vi "ControlePosicaoServo2.vi"() -> ()   [LabVIEW 2012]
uses:
  <vilib>/LabVIEW Interface for Arduino/Type Defs/Board Type.ctl
  <vilib>/LabVIEW Interface for Arduino/Type Defs/Pin Mode.ctl
  <vilib>/Utility/file.llb/Read From Spreadsheet File (I64).vi
  <vilib>/LabVIEW Interface for Arduino/LabVIEW Interface for Arduino.lvlib
panel:
  out "?":cluster{"Referencia":dbl, "Atual":dbl}(graph)
  in  "Limpar Arquivo":bool
  in  "Gravar Posição KNOOB":bool
  out "Index":u32
  out "Comeco do Timer 2":i32
  in  "Comeco do Timer":i32
  in  "Ligar Controle":bool
  out "Voltage":dbl(knob) scale=0.0..5.0
  out "Sequencia":i64[](array[numeric])
  in  "Comeco do Arquivo":i32
  out "Elemento do Arquivo":i64
  in  "file path (dialog if empty)":path
  in  "TXT    KNOOB":bool
  out "PWM2":i32
  out "PWM1":i32
  out "Erro":dbl
  in  "Referencia":dbl(knob) scale=0.0..180.0
  out "Referencia":dbl(knob) scale=0.0..180.0
  in  "stop":bool
  out "Atual":dbl(knob) scale=0.0..180.0
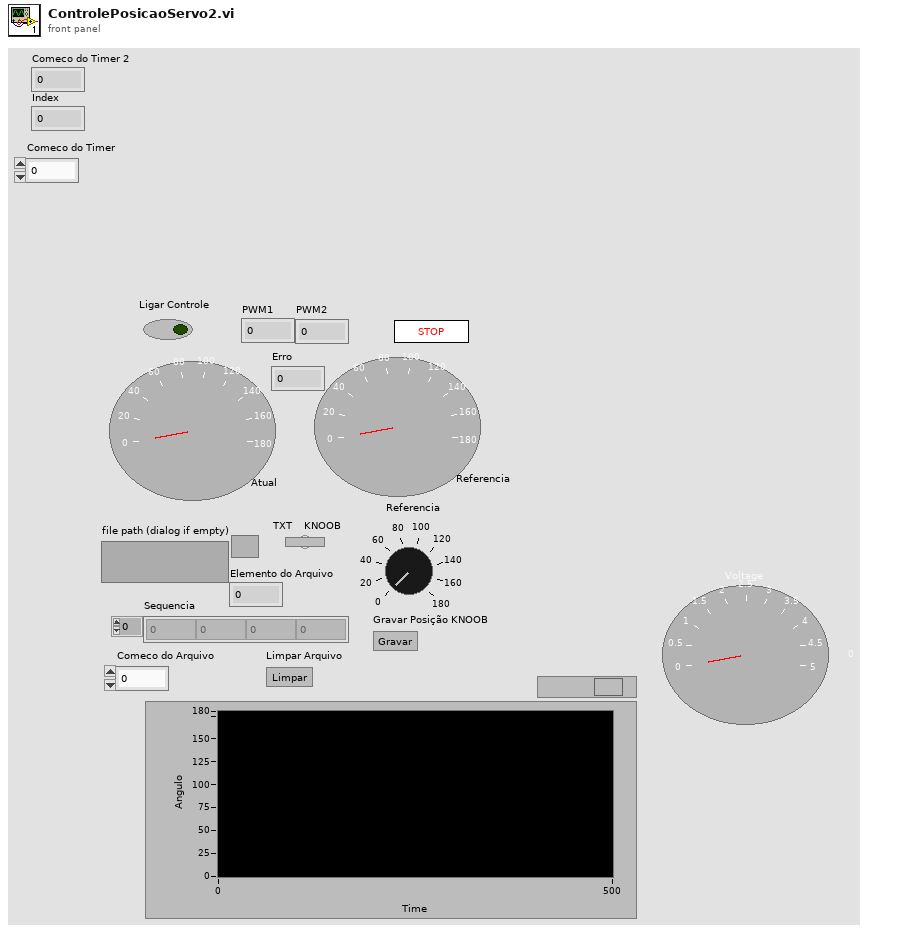
[diagram p1: front panel]
types:
  T1 = typedef "LabVIEW Interface for Arduino.lvlib/Board Type.ctl" = enum16{"Uno", "Dimuelanove w/Atmega 328", "Mega 2560"}
  T2 = typedef "LabVIEW Interface for Arduino.lvlib/Arduino Resource.ctl" = cluster{"VISA resource":refnum<visa-resource-name>, "Board Type":T1, "Connection Type":enum8{"USB / Serial"}, "Bytes Per Packet (15)":u8}
  T3 = typedef "LabVIEW Interface for Arduino.lvlib/Pin Mode.ctl" = enum8{"Input", "Output"}
  T4 = enum16{"open", "replace", "create", "open or create", "replace or create", "replace or create with confirmation"}
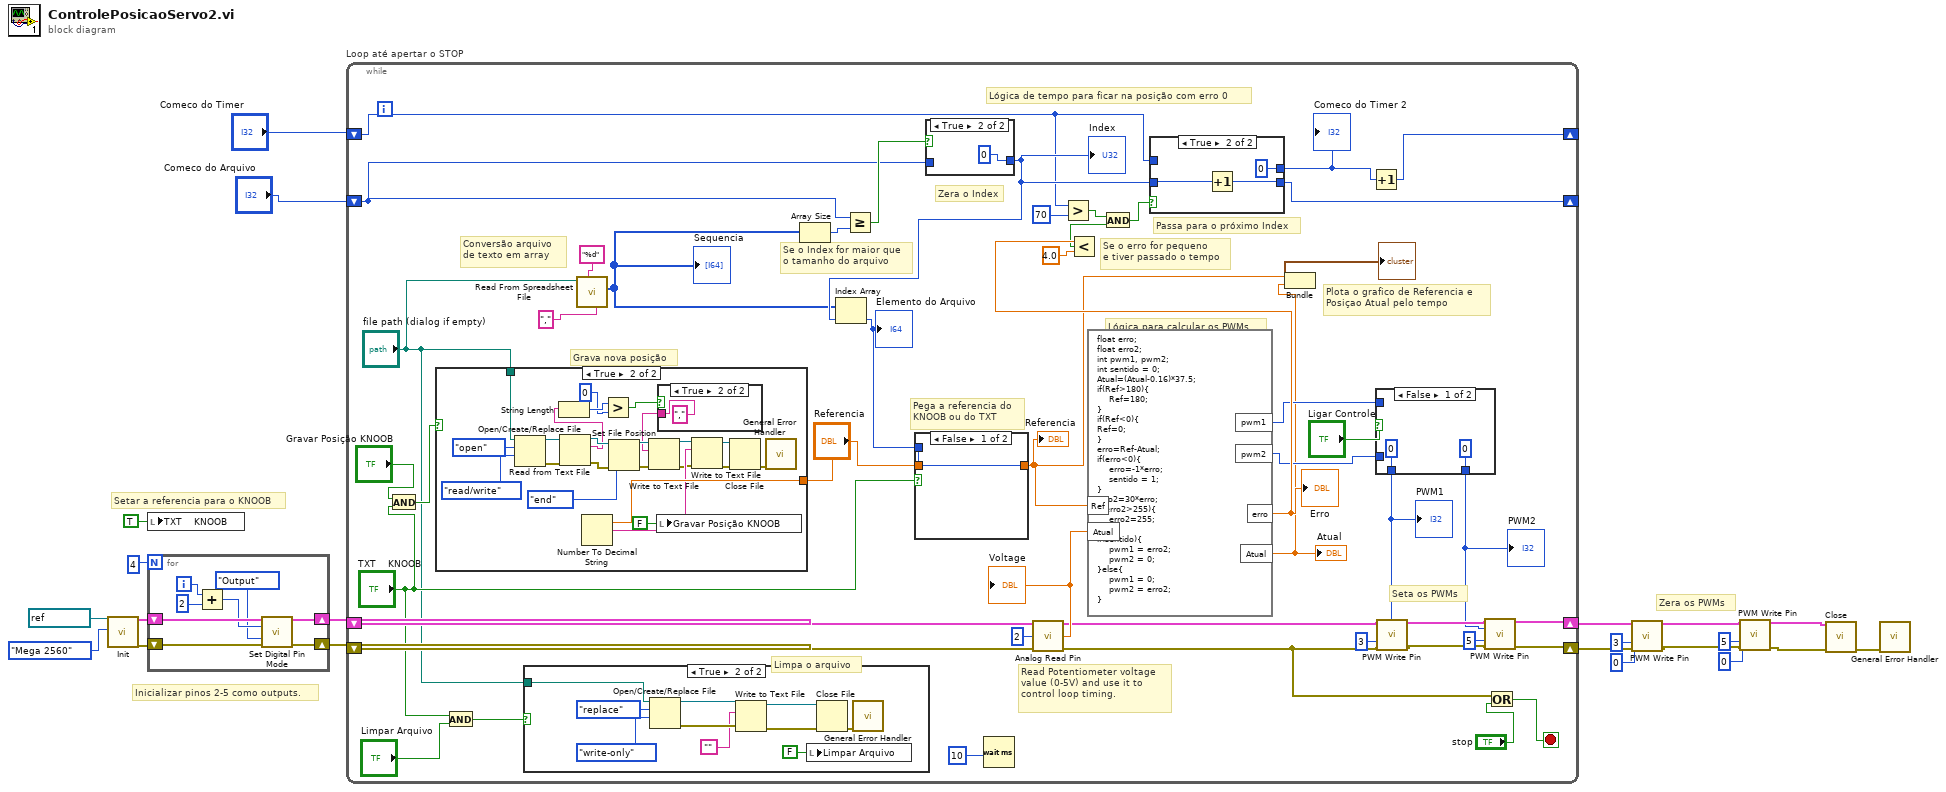
[diagram p0: block diagram]
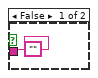
[diagram p4: hidden frame]
diagram:
  # "Zera os PWMs"
  # "Setar a referencia para o KNOOB"
  # "Inicializar pinos 2-5 como outputs."
  n1 = call <vilib>:"Init.vi"("VISA resource"=refnum<visa-resource-name> "COM6", "Board Type (Uno)"=Board_Type."Mega 2560") -> ("Arduino Resource"=w20:T2, "error out"=w21:errorcluster)  [unwired: 16 in]
  n2 = local write "TXT    KNOOB"(TRUE ("TXT    KNOOB")) -> ()
  n3 = for {
    N: 4 -> [_]
    shift-right: [w27] -> w19
    shift-left: w20 -> [w28]
    shift-right: [w26] -> w18
    shift-left: w21 -> [w29]
    i -> [w25]
    n4 = Add(x=w25, y=2) -> (x+y=w23:i32)
    n5 = call <vilib>:"Set Digital Pin Mode.vi"("Arduino Resource"=w28, "Digital I/O Pin"=w23, "Pin Mode (Input)"=Pin_Mode."Output", "error in"=w29) -> ("Arduino Resource"=w27:T2, "error out"=w26:errorcluster)  [unwired: 10 in]
  }
  n6 = while "Loop até apertar o STOP" {
    shift-right: [w69] -> w7
    shift-left: w19 -> [w76]
    shift-right: [w68] -> w6
    shift-left: w18 -> [w77]
    shift-right: [w62] -> _
    shift-left: "Comeco do Arquivo" -> [w56]
    shift-right: [w43] -> _
    shift-left: "Comeco do Timer" -> [w49]
    stop <- w63 stop-if-true
    # "Limpa o arquivo"
    # "Grava nova posição"
    # "Pega a referencia do \nKNOOB ou do TXT"
    # "Lógica para calcular os PWMs"
    # "Seta os PWMs"
    # "Plota o grafico de Referencia e \nPosiçao Atual pelo tempo"
    # "Passa para o próximo Index"
    # "Se o erro for pequeno\ne tiver passado o tempo"
    # "Zera o Index"
    # "Se o Index for maior que\no tamanho do arquivo"
    # "Conversão arquivo \nde texto em array"
    # "Lógica de tempo para ficar na posição com erro 0"
    # "Read Potentiometer voltage value (0-5V) and use it to control loop timing."
    n7 = And(x="Gravar Posição KNOOB", y="TXT    KNOOB") -> (x .and. y?=w37:bool)
    n8 = case shown="True" w37 {
      tunnel: "file path (dialog if empty)" -> [_ w107]
      tunnel: "Referencia" -> [_ w103]
      frame False {
      }
      frame True {
        n9 = Open/Create/Replace File(file path (use dialog)=w107, operation (0:open)=T4."open", access (0:read/write)=enum16{"read/write", "read-only", "write-only"}."read/write") -> (refnum out=w96:refnum<file>, error out=w95:errorcluster)  [unwired: 3 in, 1 out]
        n10 = Read from Text File(file (use dialog)=w96, error in=w95) -> (refnum out=w94:refnum<file>, text=w92:string, error out=w93:errorcluster)  [unwired: 2 in, 1 out]
        n11 = String Length(string=w92) -> (length=w90:i32)
        n12 = Number To Decimal String(number=w103) -> (decimal integer string=w102:string)  [unwired: 1 in]
        n13 = Greater?(x=w90, y=0 ("x")) -> (0:w88:bool)
        n14 = Set File Position(refnum=w94, from (0:start)=enum16{"start", "end", "current"}."end", error in=w93) -> (refnum out=w100:refnum<file>, error out=w99:errorcluster)  [unwired: 1 in]
        n15 = local write "Gravar Posição KNOOB"(FALSE ("Gravar Posição KNOOB")) -> ()
        n16 = case shown="True" w88 {
          tunnel: ["" "," ("text")] -> w91
          frame False {
          }
          frame True {
          }
        }
        n17 = Write to Text File(file (use dialog)=w100, text=w91, error in=w99) -> (refnum out=w101:refnum<file>, error out=w98:errorcluster)  [unwired: 1 in, 1 out]
        n18 = Write to Text File(file (use dialog)=w101, text=w102, error in=w98) -> (refnum out=w110:refnum<file>, error out=w108:errorcluster)  [unwired: 1 in, 1 out]
        n19 = Close File(refnum=w110, error in=w108) -> (error out=w109:errorcluster)  [unwired: 1 out]
        n20 = call <vilib>:"General Error Handler.vi"("error in (no error)"=w109) -> ()  [unwired: 10 in, 5 out]
      }
    }
    n21 = And(x="TXT    KNOOB", y="Limpar Arquivo") -> (x .and. y?=w34:bool)
    n22 = case shown="True" w34 {
      tunnel: "file path (dialog if empty)" -> [_ w84]
      frame False {
      }
      frame True {
        n23 = Open/Create/Replace File(file path (use dialog)=w84, operation (0:open)=T4."replace", access (0:read/write)=enum16{"read/write", "read-only", "write-only"}."write-only") -> (refnum out=w81:refnum<file>, error out=w80:errorcluster)  [unwired: 3 in, 1 out]
        n24 = Write to Text File(file (use dialog)=w81, text="", error in=w80) -> (refnum out=w83:refnum<file>, error out=w82:errorcluster)  [unwired: 1 in, 1 out]
        n25 = local write "Limpar Arquivo"(FALSE ("Limpar Arquivo")) -> ()
        n26 = Close File(refnum=w83, error in=w82) -> (error out=w87:errorcluster)  [unwired: 1 out]
        n27 = call <vilib>:"General Error Handler.vi"("error in (no error)"=w87) -> ()  [unwired: 10 in, 5 out]
      }
    }
    n28 = call-poly <vilib>:"Read From Spreadsheet File.vi"("delimiter (\\t)"="," ("delimiter (\\t)"), "format (%d)"="%d", "file path (dialog if empty)"="file path (dialog if empty)") -> ("first row"=w40:i64[])  [unwired: 4 in, 4 out]
    "Sequencia" <- w40
    n29 = Array Size(array=w40) -> (size(s)=w58:i32)
    n30 = Greater Or Equal?(x=w56, y=w58) -> (x >= y?=w57:bool)
    n31 = case shown="True" w57 {
      tunnel: [w117 u32 0 ("milliseconds to wait")] -> w50
      tunnel: w56 -> [w117 _]
      frame False {
      }
      frame True {
      }
    }
    "Index" <- w50
    n32 = Index Array(array=w40, index=w50) -> (element=w61:i64)
    "Elemento do Arquivo" <- w61
    n33 = case shown="False" "TXT    KNOOB" {
      tunnel: "Referencia" -> [_ w120]
      tunnel: [w119 w120] -> w32
      tunnel: w61 -> [w119 _]
      frame False {
      }
      frame True {
      }
    }
    "Referencia" <- w32
    n34 = Wait (ms)(milliseconds to wait=u32 10) -> ()  [unwired: 1 out]
    n35 = call <vilib>:"Analog Read Pin.vi"("Arduino Resource"=w76, "Analog Input Pin (0)"=u8 2, "error in"=w77) -> ("Arduino Resource"=w73:T2, "Voltage"=w74:dbl, "error out"=w64:errorcluster)  [unwired: 10 in]
    "Voltage" <- w74
    n36 = Greater?(x=w49, y=70) -> (0:w45:bool)
    n37 = formula code="float erro;\nfloat erro2;\nint pwm1, pwm2;\nint sentido = 0;\nAtual=(Atual-0.16)*37.5;\nif(Ref>180){\n    Ref=180;\n}\nif(Ref<0){\nRef=0;\n}\nerro=Ref-Atual;\nif(erro<0){\n    erro=-1*erro;\n    sentido = 1;\n}\nerro2=30*erro;\nif(erro2>255){\n    erro2=255;\n}\nif(sentido){\n    pwm1 = erro2;\n    pwm2 = 0;\n}else{\n    pwm1 = 0;\n    pwm2 = erro2;\n}"("Ref"=w32, "Atual"=w74) -> ("erro"=w60:dbl, "Atual"=w31:dbl, "pwm1"=w54:i32, "pwm2"=w53:i32)
    "Atual" <- w31
    "Erro" <- w60
    n38 = Less?(x=w60, y=4.0) -> (x < y?=w44:bool)
    n39 = And(x=w45, y=w44) -> (x .and. y?=w46:bool)
    n40 = case shown="True" w46 {
      tunnel: w50 -> [w122 w125]
      tunnel: [w122 w124] -> w62
      tunnel: [w121 0 ("Comeco do Timer")] -> w47
      tunnel: w49 -> [w121 _]
      frame False {
      }
      frame True {
        n41 = Increment(x=w125) -> (x+1=w124:u32)
      }
    }
    "Comeco do Timer 2" <- w47
    n42 = Bundle("Referencia"=w32, "Atual"=w31) -> (→"?":cluster{"Referencia":dbl, "Atual":dbl})  [unwired: 1 in]
    n43 = Increment(x=w47) -> (x+1=w43:i32)
    n44 = case shown="False" "Ligar Controle" {
      tunnel: w54 -> [_ w116]
      tunnel: [0 w116] -> w51
      tunnel: w53 -> [_ w115]
      tunnel: [0 w115] -> w52
      frame False {
      }
      frame True {
      }
    }
    "PWM1" <- w51
    "PWM2" <- w52
    n45 = call <vilib>:"PWM Write Pin.vi"("Arduino Resource"=w73, "Duty Cycle (0 - 255)"=w51, "PWM Pin (3)"=u8 3, "error in"=w64) -> ("Arduino Resource"=w71:T2, "error out"=w70:errorcluster)  [unwired: 10 in]
    n46 = call <vilib>:"PWM Write Pin.vi"("Arduino Resource"=w71, "Duty Cycle (0 - 255)"=w52, "PWM Pin (3)"=u8 5, "error in"=w70) -> ("Arduino Resource"=w69:T2, "error out"=w68:errorcluster)  [unwired: 10 in]
    n47 = Or(x=w64, y="stop") -> (x .or. y?=w63:bool)
  }
  n48 = call <vilib>:"PWM Write Pin.vi"("Arduino Resource"=w7, "Duty Cycle (0 - 255)"=u8 0, "PWM Pin (3)"=u8 3, "error in"=w6) -> ("Arduino Resource"=w10:T2, "error out"=w9:errorcluster)  [unwired: 10 in]
  n49 = call <vilib>:"PWM Write Pin.vi"("Arduino Resource"=w10, "Duty Cycle (0 - 255)"=u8 0, "PWM Pin (3)"=u8 5, "error in"=w9) -> ("Arduino Resource"=w4:T2, "error out"=w5:errorcluster)  [unwired: 10 in]
  n50 = call <vilib>:"Close.vi"("Arduino Resource"=w4, "error in"=w5) -> ("error out"=w15:errorcluster)  [unwired: 13 in]
  n51 = call <vilib>:"General Error Handler.vi"("error in (no error)"=w15) -> ()  [unwired: 10 in, 5 out]
